vi "Detect Circles - Copy.vi"(4 "Image 3":T1(plugin-control), 5 "Color Plane":i32(ring)=2 items=["Red", "Green", "Blue", "Hue", "Saturation", "Luminance", "Value", "Intensity"]) -> (0 "Circles 2":cluster{"x":dbl, "y":dbl, "r":dbl}[](array[cluster]), 1 "Image 4":T1(plugin-control), 2 "Circles":cluster{"x":dbl, "y":dbl, "r":dbl}[](array[cluster]))   [LabVIEW 2018]
panel:
  out "Circles Calibrated (Shape Detection 1)":T2(array[cluster]) {"Position"."Y" format="%.2f"; "Position"."X" format="%.2f"}
  out "Circle":T2(array[cluster]) {"Position"."Y" format="%.2f"; "Position"."X" format="%.2f"}
  out "Ellipses":T3(array[cluster])
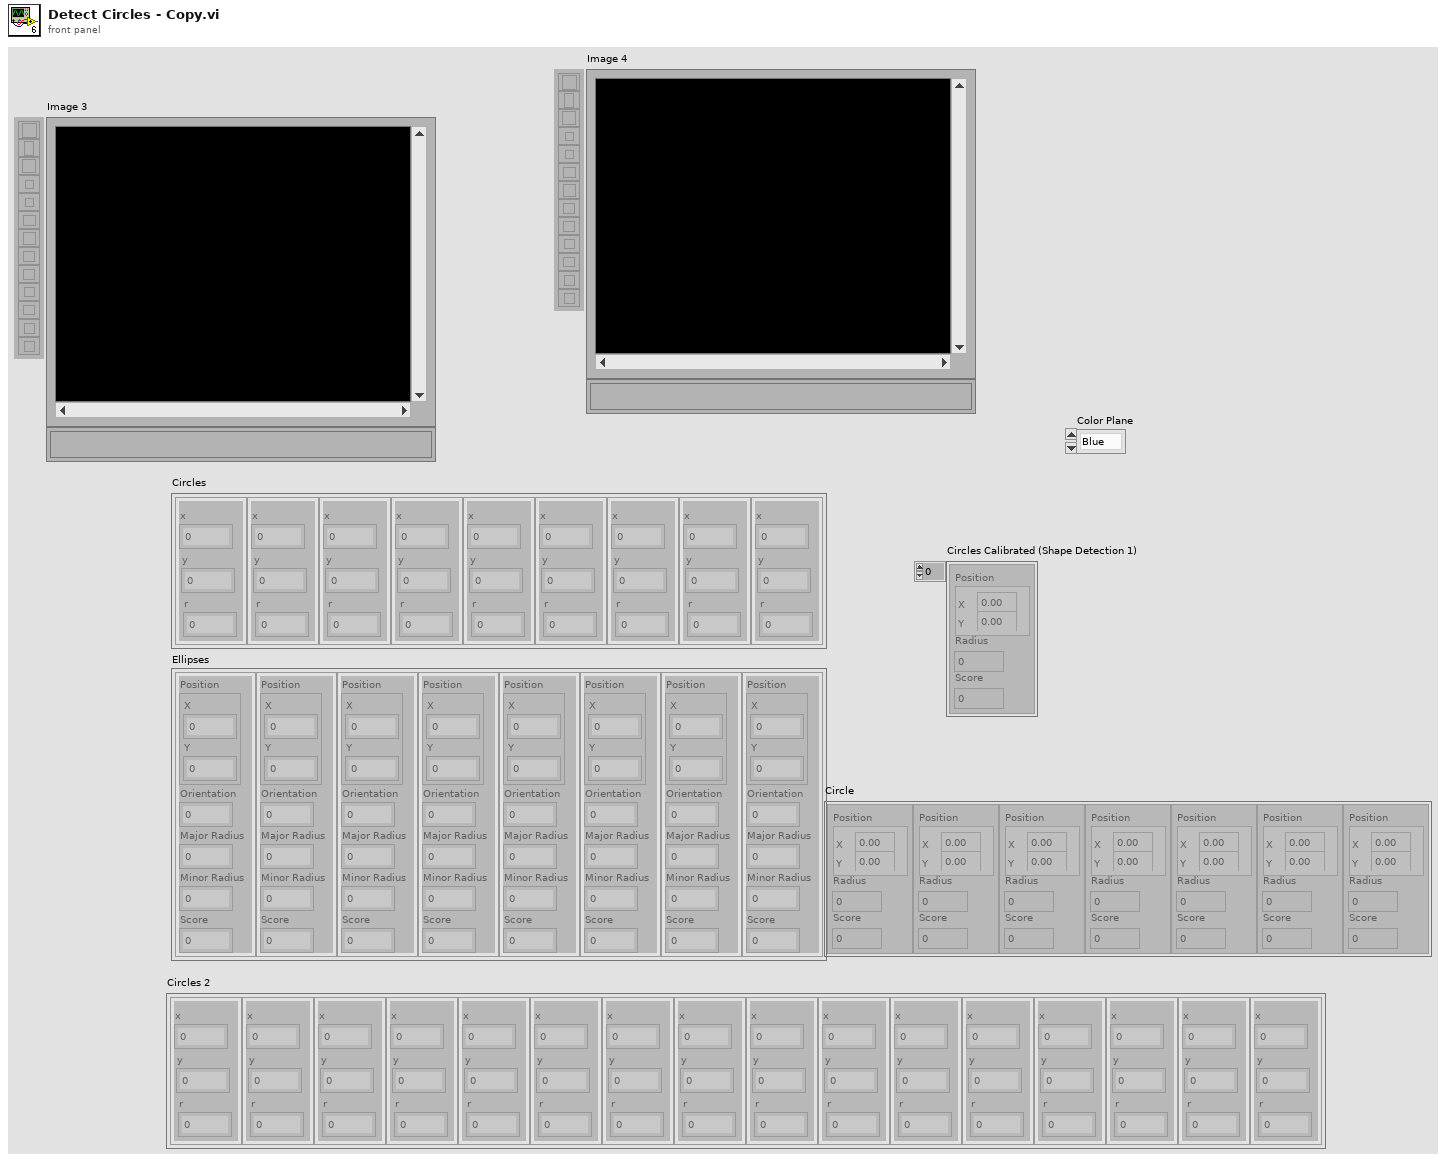
[diagram p1: front panel]
types:
  T1 = typedef "IMAQ Image.ctl" = refnum<image>
  T2 = cluster{"Position":cluster{"X":sgl, "Y":sgl}, "Radius":dbl, "Score":dbl}[]
  T3 = cluster{"Position":cluster{"X":sgl, "Y":sgl}, "Orientation":dbl, "Major Radius":dbl, "Minor Radius":dbl, "Score":dbl}[]
  T4 = cluster{"Position":cluster{"X":sgl, "Y":sgl}, "Orientation":dbl, "Major Radius":dbl, "Minor Radius":dbl, "Score":dbl}
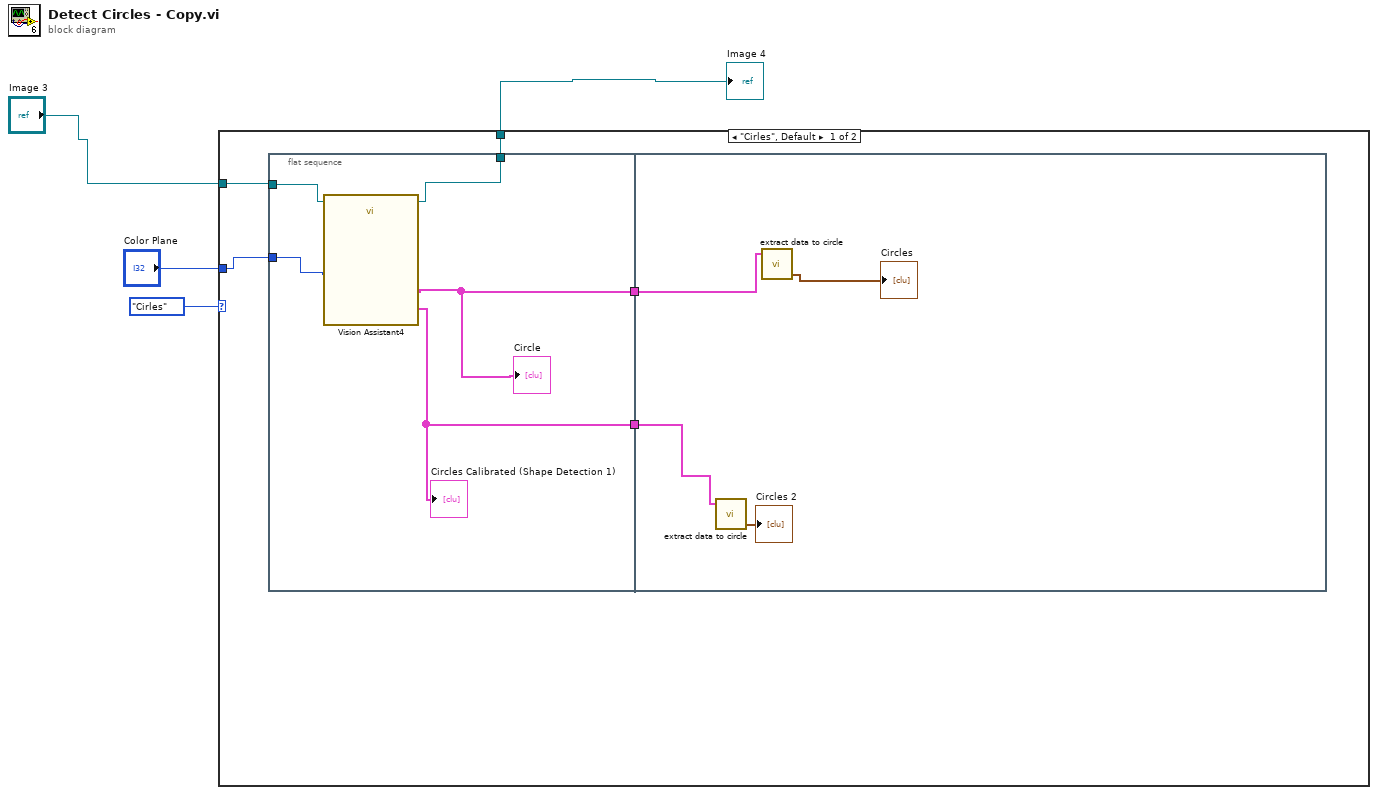
[diagram p0: block diagram]
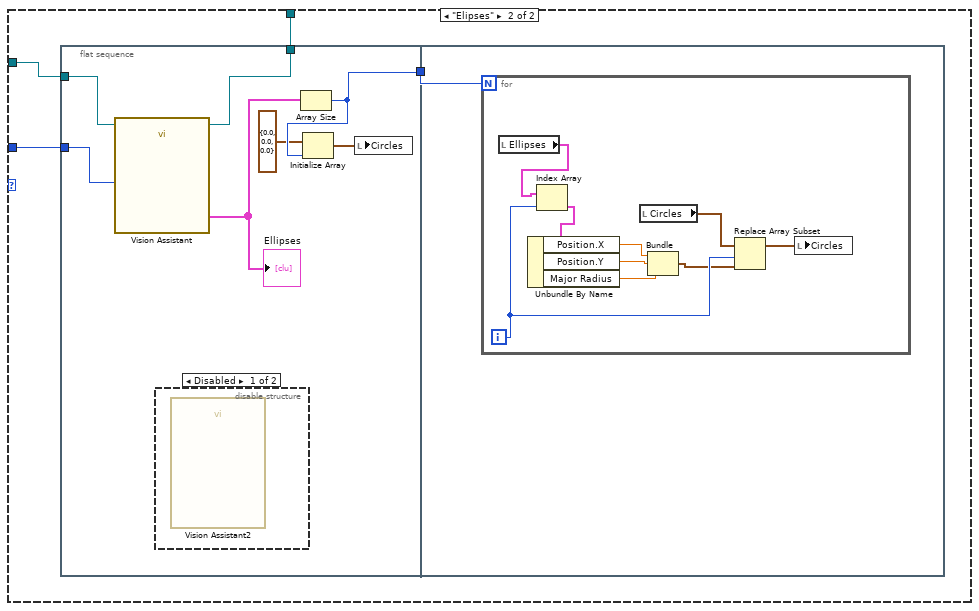
[diagram p2: hidden frame]
diagram:
  n1 = case shown="\"Cirles\", Default" enum16{"Cirles", "Elipses", ""}."Cirles" ("Shape") {
    tunnel: [w8 w22] -> w1
    tunnel: "Image 3" -> [w9 w21]
    tunnel: "Color Plane" -> [w7 w19]
    frame "Cirles", Default {
      n2 = flat-sequence {
        tunnel: [w13] -> w8
        tunnel: w9 -> [w10]
        tunnel: w7 -> [w14]
        tunnel: [w12] -> w6
        tunnel: [w11] -> w5
        tunnel: w6 -> [w16]
        tunnel: w5 -> [w15]
        frame #0 {
          n3 = call "Vision Assistant4"("Image In"=w10, "Color Plane (Color Plane Extraction 1)"=w14) -> ("Image Out"=w13:T1, "Circles (Shape Detection 1)"=w12:T2, "Circles Calibrated (Shape Detection 1)"=w11:T2)  [unwired: 22 in, 1 out]
          "Circle" <- w12
          "Circles Calibrated (Shape Detection 1)" <- w11
        }
        frame #1 {
          n4 = call "extract data to circle.vi"("Circles (Shape Detection 1)"=w15) -> ("Circles"=→"Circles 2":cluster{"x":dbl, "y":dbl, "r":dbl}[])  [unwired: 2 in, 2 out]
          n5 = call "extract data to circle.vi"("Circles (Shape Detection 1)"=w16) -> ("Circles"=→"Circles":cluster{"x":dbl, "y":dbl, "r":dbl}[])  [unwired: 2 in, 2 out]
        }
      }
    }
    frame "Elipses" {
      n6 = flat-sequence {
        tunnel: [w25] -> w22
        tunnel: w21 -> [w26]
        tunnel: [w28] -> w20
        tunnel: w19 -> [w23]
        tunnel: w20 -> [w30]
        frame #0 {
          n7 = call "Vision Assistant"("Image In"=w26, "Color Plane (Color Plane Extraction 1)"=w23) -> ("Image Out"=w25:T1, "Ellipses (Shape Detection 1)"=w24:T3)  [unwired: 23 in, 1 out]
          "Ellipses" <- w24
          n8 = disable-structure shown="Disabled" {
            frame Disabled {
              n9 = call "Vision Assistant2"() -> ()  [unwired: 25 in, 3 out]
            }
            frame Enabled {
            }
          }
          n10 = Array Size(array=w24) -> (size(s)=w28:i32)
          n11 = Initialize Array(cluster{"x":dbl, "y":dbl, "r":dbl} {"x"=0.0, "y"=0.0, "r"=0.0} ("circle"), w28) -> (w29:cluster{"x":dbl, "y":dbl, "r":dbl}[])
          n12 = local write "Circles"(w29) -> ()
        }
        frame #1 {
          n13 = for {
            N: w30 -> [_]
            i -> [w33]
            n14 = local read "Ellipses"() -> (w39:T3)
            n15 = Index Array(array=w39, index=w33) -> (element=w38:T4)
            n16 = Unbundle By Name(w38) -> ("Position.X"=w37:sgl, "Position.Y"=w36:sgl, "Major Radius"=w35:dbl)
            n17 = local read "Circles"() -> (w34:cluster{"x":dbl, "y":dbl, "r":dbl}[])
            n18 = Bundle("X"=w37, "Y"=w36, "Major Radius"=w35) -> (w32:cluster{"X":sgl, "Y":sgl, "Major Radius":dbl})  [unwired: 1 in]
            n19 = Replace Array Subset(array=w34, new element=w32, index=w33) -> (w31:cluster{"x":dbl, "y":dbl, "r":dbl}[])
            n20 = local write "Circles"(w31) -> ()
          }
        }
      }
    }
  }
  "Image 4" <- w1
